vi "Curtin1_NewTest.vi"(9 "Template name":string, 11 "Settings":T2={"Name of test"="", "Date"=timestamp(0 s since 1904-01-01), "Location"="", "Default Template"="", "Soundcard"="", "resolution"=32, "Sampling rate"=48000, "Ch1 Gain "=25.0, "Ch2 Gain"=10.0, "Sample time (s)"=0.3, "Pre-trigger (s)"=0.01, "Hammer Threshold"=10.0, "Positions"=12, "Taps/Position"=5, "Set Names"="", "Freq resolution"=10.0, "Hammer cutoff"=0.0, "Mic cutoff"=0.0, "Double bounce "=0.0, "Hammer Cal"=10.0, "dB Offset"=0.0, "Accel Cal"=10.0, "Vibrometer Cal"=0.0, "Mic Cal"=0.0, "Output"=2, "Voltage Cal"=0.01, "Vibrometer Port"="ASRL27::INSTR", "Range"=4, "High Pass"=2, "Bandwidth"=4, "X Range"=[{"Minimum"=200.0, "Maximum"=10000.0, "Increment"=10.0, "Minor Increment"=100.0, "Start"=200.0}, {"Minimum"=0.0, "Maximum"=0.05, "Increment"=0.025, "Minor Increment"=0.0025, "Start"=0.0}, {"Minimum"=0.0, "Maximum"=0.3, "Increment"=0.1, "Minor Increment"=0.01, "Start"=0.0}, {"Minimum"=200.0, "Maximum"=10000.0, "Increment"=10.0, "Minor Increment"=100.0, "Start"=1000.0}], "Y Range"=[{"Minimum"=-25.0, "Maximum"=0.0, "Increment"=5.0, "Minor Increment"=1.0, "Start"=-25.0}, {"Minimum"=-0.01, "Maximum"=0.1, "Increment"=0.02, "Minor Increment"=0.005, "Start"=0.0}, {"Minimum"=-0.1, "Maximum"=0.1, "Increment"=0.05, "Minor Increment"=0.01, "Start"=-0.1}, {"Minimum"=-35.0, "Maximum"=5.0, "Increment"=2.0, "Minor Increment"=0.5, "Start"=-34.0}], "dB Spread"=0.0, "Trigger"=0, "Ch_1"=25, "Ch_2"=25, "flip?"=FALSE, "60Hz"=FALSE, "Time Offset"=0.0, "Piezo Cal"=0.0, "Default Notes"=""} {"Ch_2" min=1 step=1; "Ch_1" min=1 max=100 step=1; "Trigger" items=["Hammer (force)", "Self-tap", "Spacebar"]; "Bandwidth" items=["1 kHz"=1, "5 kHz"=5, "10 kHz"=10, "25 kHz"=25, "50 kHz"=50, "100 kHz"=100]; "High Pass" items=["Off", "13 Hz", "104 Hz"]; "Range" items=["10 mm/s"=1, "20 mm/s"=2, "50 mm/s"=5, "100 mm/s"=10, "200 mm/s"=20, "500 mm/s"=50, "1 m/s"=100, "2 m/s"=200]; "Output" items=["Accelerometer", "Speed (from acceleration)", "Microphone", "Vibrometer"]; "Voltage Cal" format="%#_13g"; "Ch2 Gain" format="%#_13g"; "Ch1 Gain" format="%#_13g"; "Double bounce" min=0.0; "Mic cutoff" min=0.0 format="%#_4g"; "Hammer cutoff" min=0.0 format="%#_4g"; "Freq resolution" min=0.0; "Pre-trigger (s)" format="%#_13g"; "Date" format="%<%H:%M\n%d/%m/%y>T"; "resolution" items=["16 bit"=16, "24 bit"=24, "32 bit"=32]; "Sampling rate" items=["22050 samp/s"=22050, "44100 samp/s"=44100, "48000 samp/s"=48000]}) -> (2 "Success":bool, 3 "Settings Out":T1={"Name of test"="", "Date"=timestamp(0 s since 1904-01-01), "Location"="", "Template"="", "Soundcard"="", "resolution"=32, "Sampling rate"=48000, "Ch1 Gain "=25.0, "Ch2 Gain"=10.0, "Sample time (s)"=0.3, "Pre-trigger (s)"=0.01, "Hammer Threshold"=10.0, "Positions"=12, "Taps/Position"=5, "Set Names"="", "Freq resolution"=10.0, "Hammer cutoff"=0.0, "Mic cutoff"=0.0, "Double bounce "=0.0, "Hammer Cal"=10.0, "dB Offset"=0.0, "Accel Cal"=10.0, "Vibrometer Cal"=0.0, "Mic Cal"=0.0, "Output"=2, "Voltage Cal"=0.01, "Vibrometer Port"="ASRL27::INSTR", "Range"=4, "High Pass"=2, "Bandwidth"=4, "X Range"=[], "Y Range"=[], "dB Spread"=0.0, "Trigger"=0, "Ch_1"=25, "Ch_2"=25, "flip?"=FALSE, "60Hz"=FALSE, "Time offset"=0.0, "Piezo Cal"=1.0, "Default Notes"=""} {"Ch_2" min=1 step=1; "Ch_1" min=1 max=100 step=1; "Trigger" items=["Hammer (force)", "Self-tap", "Spacebar"]; "Bandwidth" items=["1 kHz"=1, "5 kHz"=5, "10 kHz"=10, "25 kHz"=25, "50 kHz"=50, "100 kHz"=100]; "High Pass" items=["Off", "13 Hz", "104 Hz"]; "Range" items=["10 mm/s"=1, "20 mm/s"=2, "50 mm/s"=5, "100 mm/s"=10, "200 mm/s"=20, "500 mm/s"=50, "1 m/s"=100, "2 m/s"=200]; "Output" items=["Accelerometer", "Speed (from acceleration)", "Microphone", "Vibrometer", "Piezo"]; "Voltage Cal" format="%#_13g"; "Ch2 Gain" format="%#_13g"; "Ch1 Gain" format="%#_13g"; "Double bounce" min=0.0; "Mic cutoff" min=0.0 format="%#_4g"; "Hammer cutoff" min=0.0 format="%#_4g"; "Freq resolution" min=0.0; "Pre-trigger (s)" format="%#_13g"; "Date" format="%<%H:%M\n%d/%m/%y>T"; "resolution" items=["16 bit"=16, "24 bit"=24, "32 bit"=32]; "Sampling rate" items=["22050 samp/s"=22050, "44100 samp/s"=44100, "48000 samp/s"=48000]})   [LabVIEW 2022 SP3]
uses:
  PreferencesControl.ctl
  <vilib>/Utility/miscctls.llb/LVSelectionTypeDef.ctl
  <vilib>/Utility/error.llb/Trim Whitespace One-Sided.vi
  Mic/Mic_Global.vi
panel:
  in  "View":bool
  out "Comparison info":string
  out "String":string="Updating Vibrometer..."
  out "start":T1={"Name of test"="", "Date"=timestamp(0 s since 1904-01-01), "Location"="", "Template"="", "Soundcard"="", "resolution"=0, "Sampling rate"=0, "Ch1 Gain "=25.0, "Ch2 Gain"=10.0, "Sample time (s)"=0.0, "Pre-trigger (s)"=0.0, "Hammer Threshold"=0.0, "Positions"=0, "Taps/Position"=0, "Set Names"="", "Freq resolution"=0.0, "Hammer cutoff"=0.0, "Mic cutoff"=0.0, "Double bounce "=0.0, "Hammer Cal"=0.0, "dB Offset"=0.0, "Accel Cal"=0.0, "Vibrometer Cal"=0.0, "Mic Cal"=0.0, "Output"=0, "Voltage Cal"=1.0, "Vibrometer Port"="ASRL27::INSTR", "Range"=4, "High Pass"=2, "Bandwidth"=4, "X Range"=[], "Y Range"=[], "dB Spread"=0.0, "Trigger"=0, "Ch_1"=25, "Ch_2"=25, "flip?"=FALSE, "60Hz"=FALSE, "Time offset"=0.0, "Piezo Cal"=1.0, "Default Notes"=""} {"Ch_2" min=1 step=1; "Ch_1" min=1 max=100 step=1; "Trigger" items=["Hammer (force)", "Self-tap", "Spacebar"]; "Bandwidth" items=["1 kHz"=1, "5 kHz"=5, "10 kHz"=10, "25 kHz"=25, "50 kHz"=50, "100 kHz"=100]; "High Pass" items=["Off", "13 Hz", "104 Hz"]; "Range" items=["10 mm/s"=1, "20 mm/s"=2, "50 mm/s"=5, "100 mm/s"=10, "200 mm/s"=20, "500 mm/s"=50, "1 m/s"=100, "2 m/s"=200]; "Output" items=["Accelerometer", "Speed (from acceleration)", "Microphone", "Vibrometer", "Piezo"]; "Voltage Cal" format="%#_13g"; "Ch2 Gain" format="%#_13g"; "Ch1 Gain" format="%#_13g"; "Double bounce" min=0.0; "Mic cutoff" min=0.0 format="%#_4g"; "Hammer cutoff" min=0.0 format="%#_4g"; "Freq resolution" min=0.0; "Pre-trigger (s)" format="%#_13g"; "Date" format="%<%H:%M\n%d/%m/%y>T"; "resolution" items=["16 bit"=16, "24 bit"=24, "32 bit"=32]; "Sampling rate" items=["22050 samp/s"=22050, "44100 samp/s"=44100, "48000 samp/s"=48000]}
  in  "DAQ":bool
  out "current":string
  out "Hammer Spectrum":cluster{dbl, "df":dbl, "FFT {X}":dbl[]}[](graph)=[{0.0, "df"=1.0, "FFT {X}"=array[24000 elements]}, {0.0, "df"=40000.0, "FFT {X}"=[-20.0, -20.0]}]
  out "Hammer Data":cluster{dbl, "dt":dbl, "Y":dbl[]}[](graph)=[{0.0, "dt"=2.0833333333333333e-05, "Y"=array[14400 elements]}, {0.0, "dt"=0.0, "Y"=[]}]
  out "Microphone Data":cluster{dbl, "dt":dbl, "Y":dbl[]}[](graph)=[{0.0, "dt"=2.0833333333333333e-05, "Y"=array[14400 elements]}, {0.0, "dt"=0.0, "Y"=[]}]
  out "Average FRF":cluster{dbl, "df":dbl, dbl[]}[](graph)=[{0.0, "df"=1.0, array[24000 elements]}, {0.0, "df"=1.0, array[24000 elements]}]
  out "Vib Cover":bool
  in  "Vibrometer 2":bool
  in  "Vibrometer":bool
  in  "Save as a Template":bool
  in  "Import Template":bool
  in  "Test":bool
  in  "device:":u16(ring) items=["BuerginBase Microphone", "485B39 200083408035100798118210422", "MacBook Pro Microphone", "Reincubate", "Microsoft Teams Audio", "Jump Desktop Microphone", "Jump Desktop Audio", "ZoomAudioDevice"]
  in  "OK Button":bool
  in  "Cancel Button":bool
  in  "Instrument Notes":string
  in  "Tag List":bool
  in  "Instrument Name":string(combo)
  in  "Instrument Keywords":string
  out "File name":string
  in  "Test Name":string
  in  "Import Calib":bool
  # "New Test"
  # "Adjust default scale ranges"
  # "Adjust default scale ranges"
  # "Hz"
  # "dB"
  # "dB"
  # "sec"
  # "sec"
  # "mV/Pa"
  # "mV/m/s2"
  # "mV/mm/s"
  # "V/N"
  # "sec"
  # "sec"
  # "mV/N"
  # "a.u."
  # "a.u."
  # "sec"
  # "mV/Pa"
  # "mV/m/s2"
  # "mV/mm/s"
  # "V/N"
  # "sec"
  # "sec"
  # "mV/N"
  # "Hz"
  # "a.u."
  # "dB"
  # "a.u."
  # "dB"
  # "sec"
  # "sec"
  # "sec"
  # "Hz"
  # "dB"
  # "dB"
  # "sec"
  # "sec"
  # "mV/Pa"
  # "mV/m/s2"
  # "mV/mm/s"
  # "V/N"
  # "sec"
  # "sec"
  # "mV/N"
  # "a.u."
  # "a.u."
  # "sec"
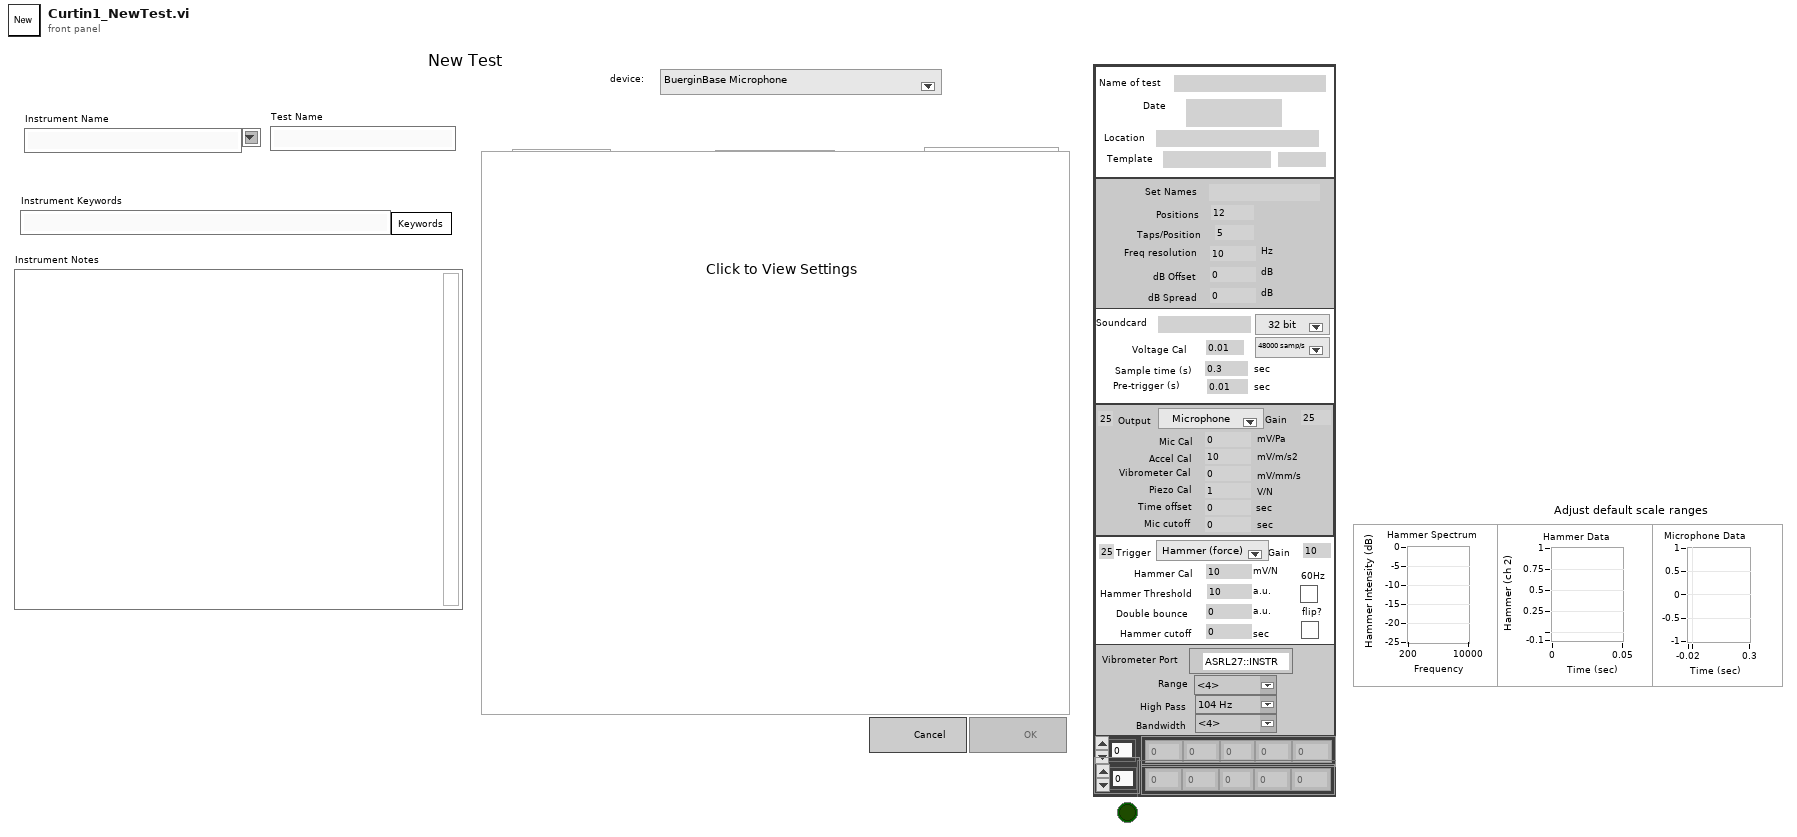
[diagram p1: front panel]
types:
  T1 = typedef "PreferencesControl.ctl" = cluster{"Name of test":string, "Date":timestamp, "Location":string, "Template":string, "Soundcard":string, "resolution":u16, "Sampling rate":u16, "Ch1 Gain ":dbl, "Ch2 Gain":dbl, "Sample time (s)":dbl, "Pre-trigger (s)":dbl, "Hammer Threshold":dbl, "Positions":i16, "Taps/Position":i16, "Set Names":string, "Freq resolution":dbl, "Hammer cutoff":dbl, "Mic cutoff":dbl, "Double bounce ":dbl, "Hammer Cal":dbl, "dB Offset":dbl, "Accel Cal":dbl, "Vibrometer Cal":dbl, "Mic Cal":dbl, "Output":u16, "Voltage Cal":dbl, "Vibrometer Port":refnum<visa-resource-name>, "Range":u16, "High Pass":u16, "Bandwidth":u16, "X Range":cluster{"Minimum":dbl, "Maximum":dbl, "Increment":dbl, "Minor Increment":dbl, "Start":dbl}[], "Y Range":cluster{"Minimum":dbl, "Maximum":dbl, "Increment":dbl, "Minor Increment":dbl, "Start":dbl}[], "dB Spread":dbl, "Trigger":u16, "Ch_1":u8, "Ch_2":u8, "flip?":bool, "60Hz":bool, "Time offset":dbl, "Piezo Cal":dbl, "Default Notes":string}
  T2 = cluster{"Name of test":string, "Date":timestamp, "Location":string, "Default Template":string, "Soundcard":string, "resolution":u16, "Sampling rate":u16, "Ch1 Gain ":dbl, "Ch2 Gain":dbl, "Sample time (s)":dbl, "Pre-trigger (s)":dbl, "Hammer Threshold":dbl, "Positions":i16, "Taps/Position":i16, "Set Names":string, "Freq resolution":dbl, "Hammer cutoff":dbl, "Mic cutoff":dbl, "Double bounce ":dbl, "Hammer Cal":dbl, "dB Offset":dbl, "Accel Cal":dbl, "Vibrometer Cal":dbl, "Mic Cal":dbl, "Output":u16, "Voltage Cal":dbl, "Vibrometer Port":refnum<visa-resource-name>, "Range":u16, "High Pass":u16, "Bandwidth":u16, "X Range":cluster{"Minimum":dbl, "Maximum":dbl, "Increment":dbl, "Minor Increment":dbl, "Start":dbl}[], "Y Range":cluster{"Minimum":dbl, "Maximum":dbl, "Increment":dbl, "Minor Increment":dbl, "Start":dbl}[], "dB Spread":dbl, "Trigger":u16, "Ch_1":u8, "Ch_2":u8, "flip?":bool, "60Hz":bool, "Time Offset":dbl, "Piezo Cal":dbl, "Default Notes":string}
  T3 = enum8{"Enabled", "Disabled", "Disabled and Grayed Out"}
  T4 = typedef "LVSelectionTypeDef.ctl" = cluster{"Selection Start":u32, "Selection End":u32}
  T5 = typedef "LVRangeTypeDef.ctl" = cluster{"Minimum":dbl, "Maximum":dbl, "Increment":dbl, "Minor Increment":dbl, "Start":dbl}
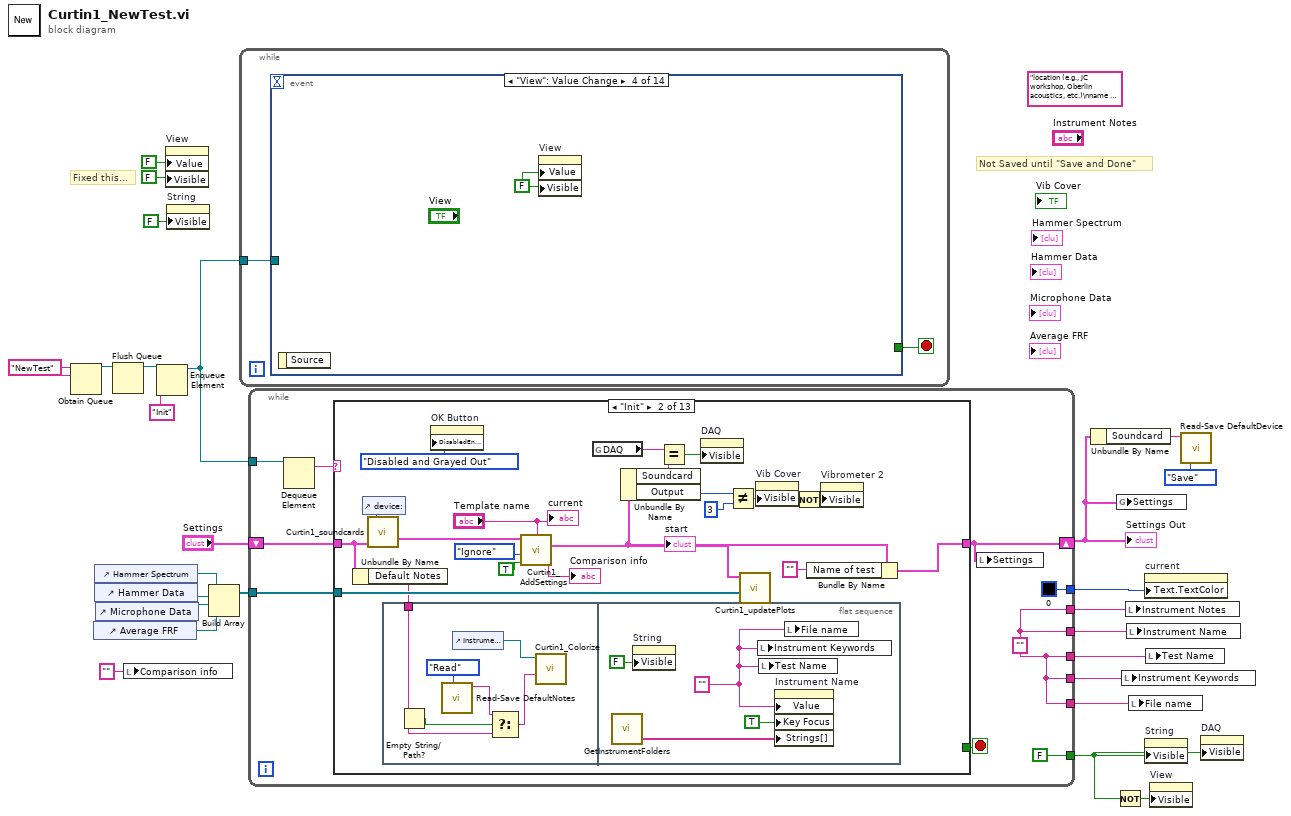
[diagram p0: block diagram]
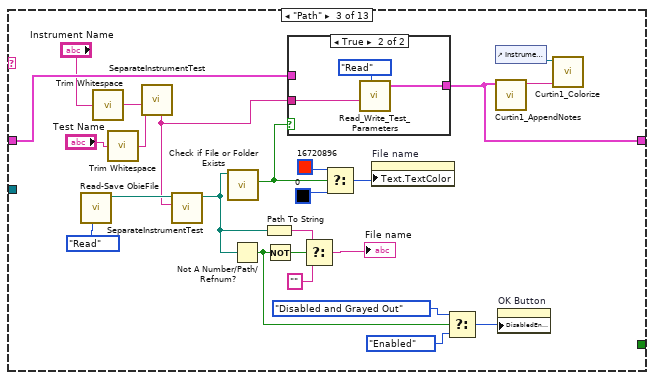
[diagram p3: hidden frame]
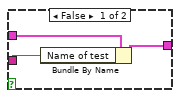
[diagram p4: hidden frame]
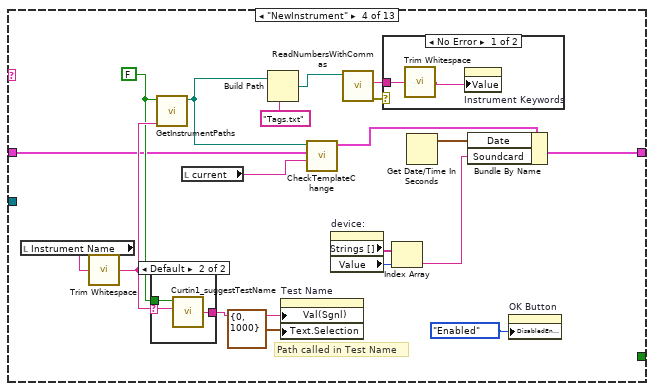
[diagram p5: hidden frame]
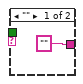
[diagram p7: hidden frame]
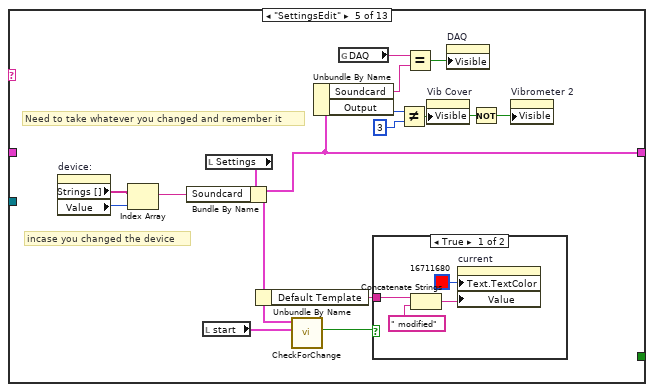
[diagram p8: hidden frame]
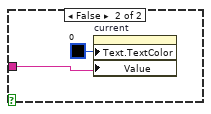
[diagram p9: hidden frame]
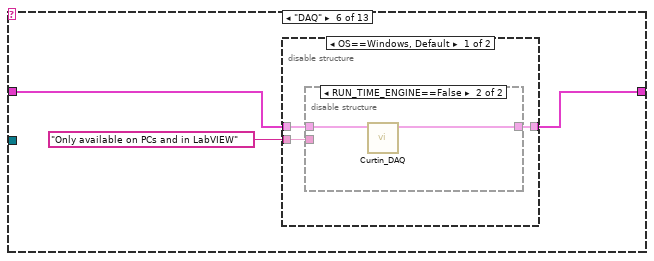
[diagram p10: hidden frame]
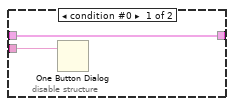
[diagram p11: hidden frame]
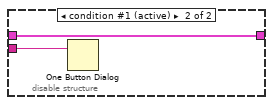
[diagram p12: hidden frame]
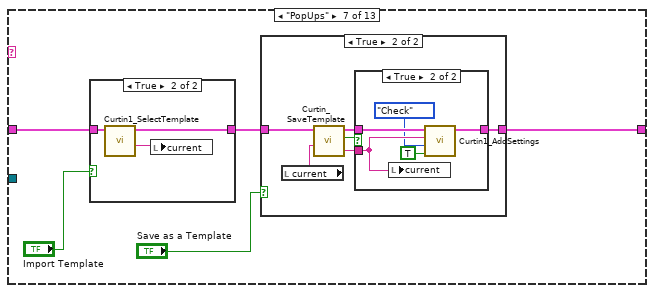
[diagram p13: hidden frame]
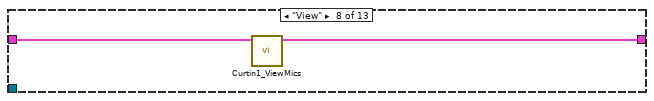
[diagram p17: hidden frame]
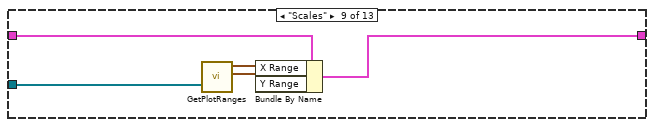
[diagram p18: hidden frame]
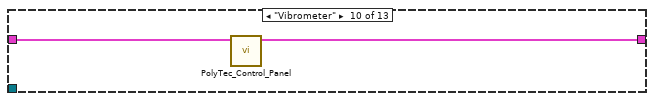
[diagram p19: hidden frame]
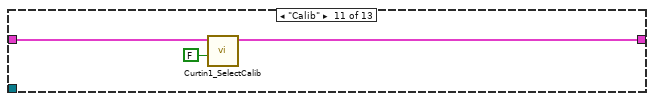
[diagram p20: hidden frame]
diagram:
  (unwired) "location (e.g., JC workshop, Oberlin acoustics, etc.)\nname of experiment (if applicable) \nnames of researchers\n\nInstrument Information:\ninstrument (e.g., violin, viola, cello, guitar, mandolin, etc.) \nmodel (e.g., Titian Strad, Guadagnini, personal, etc.) \nmaker name\nmaker ID (e.g., serial number)\nyear built (4 digits)\ncountry of origin \nsession (e.g. Oberlin 2017, VSA 2008) \nmaking school (e.g. Old Italian) \n\nMeasurement Information:\ntype (Radiation, admittance, modal analysis, taptones, etc.) \nprotocol (HV24, etc.)\n" ("Notes")
  w26 = "NewTest" ("name (unnamed)")
  # "Fixed this..."
  # "Not Saved until \"Save and Done\""
  n1 = Obtain Queue(name (unnamed)=w26, element data type=w26) -> (queue out=w3:refnum<queue>)  [unwired: 3 in, 2 out]
  n2 = control-ref of="Average FRF"() -> (w14:refnum<vi>)
  n3 = control-ref of="Hammer Spectrum"() -> (w17:refnum<vi>)
  n4 = control-ref of="Hammer Data"() -> (w16:refnum<vi>)
  n5 = control-ref of="Microphone Data"() -> (w15:refnum<vi>)
  n6 = Flush Queue(queue=w3) -> (queue out=w2:refnum<queue>)  [unwired: 1 in, 2 out]
  n7 = local write "Comparison info"("" ("Comparison info")) -> ()
  n8 = Enqueue Element(queue=w2, element="Init") -> (queue out=w24:refnum<queue>)  [unwired: 2 in, 2 out]
  n9 = property on="View" class="Bool (strict)"("Value"=FALSE ("View"), "Visible"=FALSE) -> ()  [unwired: 2 in, 2 out]
  n10 = property on="String" class="Str"("Visible"=FALSE) -> ()  [unwired: 2 in, 2 out]
  n11 = Build Array(w17, w16, w15, w14) -> (w13:refnum<vi>[])
  n12 = while {
    tunnel: w24 -> [w27]
    stop <- w28 stop-if-true
    n13 = event shown="[3] \"View\": Value Change" {
      selector: _ -> [_ _ _ _ _ _ _ _ _ _ _ _ _ _]
      dyn-events: _ -> [_ _ _ _ _ _ _ _ _ _ _ _ _ _]
      timeout: _ -> [_ _ _ _ _ _ _ _ _ _ _ _ _ _]
      tunnel: [_ _ _ _ _ _ _ _ _ _ _ _ TRUE _] -> w28
      tunnel: w27 -> [_ w29 w31 _ w34 w36 w38 w40 w42 w44 w46 w48 w54 _]
      event Timeout {
        n14 = event-data() -> ()  [unwired: 1 in, 3 out]
      }
      event "Test Name": Value Change {
        n15 = event-data() -> ()  [unwired: 1 in, 1 out]
        n16 = Enqueue Element(queue=w29, element="Path") -> ()  [unwired: 2 in, 3 out]
      }
      event "Settings": Value Change {
        n17 = event-data() -> ()  [unwired: 1 in, 1 out]
        n18 = Enqueue Element(queue=w31, element="SettingsEdit") -> ()  [unwired: 2 in, 3 out]
      }
      event "View": Value Change {
        w33 = FALSE ("Visible")
        n19 = event-data() -> ()  [unwired: 1 in, 1 out]
        n20 = property on="View" class="Bool (strict)"("Value"=w33, "Visible"=w33) -> ()  [unwired: 2 in, 2 out]
      }
      event "Instrument Name": Value Change {
        n21 = event-data() -> ()  [unwired: 1 in, 6 out]
        n22 = Enqueue Element(queue=w34, element="NewInstrument") -> ()  [unwired: 2 in, 3 out]
      }
      event "device:": Value Change {
        n23 = event-data() -> ()  [unwired: 1 in, 6 out]
        n24 = Enqueue Element(queue=w36, element="SettingsEdit") -> ()  [unwired: 2 in, 3 out]
      }
      event "DAQ": Value Change {
        n25 = event-data() -> ()  [unwired: 1 in, 6 out]
        n26 = Enqueue Element(queue=w38, element="DAQ") -> ()  [unwired: 2 in, 3 out]
      }
      event "Import Calib": Value Change {
        n27 = event-data() -> ()  [unwired: 1 in, 6 out]
        n28 = Enqueue Element(queue=w40, element="Calib") -> ()  [unwired: 2 in, 3 out]
      }
      event "Import Template", "Save as a Template": Value Change {
        n29 = event-data() -> ()  [unwired: 1 in, 1 out]
        n30 = Enqueue Element(queue=w42, element="PopUps") -> ()  [unwired: 2 in, 3 out]
      }
      event "Test": Value Change {
        n31 = event-data() -> ()  [unwired: 1 in, 6 out]
        n32 = Enqueue Element(queue=w44, element="View") -> ()  [unwired: 2 in, 3 out]
      }
      event "Average FRF", "Microphone Data", "Hammer Data", "Hammer Spectrum": Scale Range Change {
        n33 = event-data() -> ()  [unwired: 1 in, 8 out]
        n34 = Enqueue Element(queue=w46, element="Scales") -> ()  [unwired: 2 in, 3 out]
      }
      event "Vibrometer", "Vibrometer 2": Value Change {
        n35 = event-data() -> ()  [unwired: 1 in, 6 out]
        n36 = Enqueue Element(queue=w48, element="Vibrometer") -> ()  [unwired: 2 in, 3 out]
      }
      event Panel Close; "OK Button", "Cancel Button": Value Change {
        n37 = event-data() -> ()  [unwired: 1 in, 1 out]
        n38 = Select(t="Save and Done" ("element"), s="OK Button", f="Done" ("element")) -> (s? t:f=w51:string)
        n39 = Enqueue Element(queue=w54, element=w51) -> ()  [unwired: 2 in, 3 out]
        "Success" <- "OK Button"
      }
      event "Tag List", "Instrument Keywords": Value Change {
        n40 = event-data() -> ()  [unwired: 1 in, 1 out]
        n41 = case shown="True" "Tag List" {
          tunnel: ["" ("Tags out") w71] -> w60
          frame False {
          }
          frame True {
            n42 = call "RequestTags.vi"() -> ("Tags out"=w71:string)  [unwired: 11 in]
          }
        }
        n43 = case shown="Default" "Instrument Keywords" {
          tunnel: w60 -> [w61 w62]
          tunnel: "Instrument Keywords" -> [_ w64]
          tunnel: [w61 w63] -> w58
          frame "" {
          }
          frame Default {
            n44 = case shown="Default" w62 {
              selector: w62 -> [_ w66]
              tunnel: w64 -> [w65 w69]
              tunnel: [w65 w68] -> w63
              frame "" {
              }
              frame Default {
                n45 = Concatenate Strings(w69, "," ("string"), w66) -> (w68:string)
              }
            }
          }
        }
        n46 = call "RemoveDuplicateTags.vi"("Tags"=w58) -> ("Tag string"=w56:string)  [unwired: 9 in, 1 out]
        n47 = local write "Instrument Keywords"(w56) -> ()
      }
    }
  }
  n48 = while {
    tunnel: w24 -> [w79]
    shift-right: [w72] -> w5
    shift-left: "Settings" -> [w77]
    tunnel: [w76] -> w23
    tunnel: [w76] -> w22
    tunnel: [w76] -> w21
    tunnel: [w76] -> w20
    tunnel: [w76] -> w19
    tunnel: [FALSE ("Visible")] -> w8
    tunnel: w13 -> [w74]
    tunnel: [u32 0 ("Text.Text Colors:Text Color")] -> w12
    stop <- w78 stop-if-true
    w76 = "" ("Value (Signaling)")
    n49 = Dequeue Element(queue=w79) -> (element=w80:string)  [unwired: 2 in, 3 out]
    n50 = case shown="\"Init\"" w80 {
      tunnel: [_ _ _ _ _ _ _ _ _ _ _ TRUE TRUE] -> w78
      tunnel: w77 -> [w81 w84 w119 w149 _ w189 w203 w223 w225 w230 w233 w234 w239]
      tunnel: [w81 w100 w116 w154 w172 w188 w200 w222 w224 w229 w232 w234 w236] -> w72
      tunnel: w74 -> [_ w87 _ _ _ _ _ _ w226 _ _ _ _]
      frame Default {
      }
      frame "Init" {
        n51 = Unbundle By Name(w84) -> ("Default Notes"=w83:string)
        n52 = control-ref of="device:"() -> (w101:refnum<vi>)
        n53 = call "Curtin1_soundcards.vi"("Settings In"=w84, "device:"=w101) -> ("Settings Out"=w85:T1)  [unwired: 8 in, 1 out]
        n54 = flat-sequence {
          tunnel: w83 -> [w103]
          frame #0 {
            n55 = Empty String/Path?(string/path=w103) -> (empty?=w102:bool)
            n56 = call "Read-Save DefaultNotes.vi"("Task"=enum16{"Save", "Read"}."Read") -> ("Notes Out"=w105:string)  [unwired: 9 in, 1 out]
            n57 = control-ref of="Instrument Notes"() -> (w106:refnum<vi>)
            n58 = Select(t=w105, s=w102, f=w103) -> (s? t:f=w104:string)
            n59 = call "Curtin1_Colorize.vi"("Instrument Notes"=w104, "Text"=w106) -> ()  [unwired: 10 in]
          }
          frame #1 {
            w109 = "" ("Value (Signaling)")
            n60 = call "GetInstrumentFolders.vi"() -> ("folder names"=w111:string[])  [unwired: 11 in]
            n61 = property on="String" class="Str"("Visible"=FALSE) -> ()  [unwired: 2 in, 2 out]
            n62 = local write "Instrument Keywords"(w109) -> ()
            n63 = local write "Test Name"(w109) -> ()
            n64 = property on="Instrument Name" class="CmbBox"("Value"=w109, "Key Focus"=TRUE, "Strings[]"=w111) -> ()  [unwired: 2 in, 2 out]
            n65 = local write "File name"(w109) -> ()
          }
        }
        n66 = property on="OK Button" class="Bool"("DisabledEnum"=T3."Disabled and Grayed Out" ("Disabled")) -> ()  [unwired: 2 in, 2 out]
        n67 = call "Curtin1_AddSettings.vi"("Date?"=TRUE, "Check?"=enum16{"Ignore", "Check", "Replace"}."Ignore", "Template"="Template name", "Settings in"=w85) -> ("text"=→"Comparison info":string, "Settings Out"=w86:T1)  [unwired: 6 in]
        "start" <- w86
        n68 = global read "Mic_Global.vi" "DAQ"() -> (w93:string)
        n69 = Unbundle By Name(w86) -> ("Soundcard"=w92:string, "Output"=w98:u16)
        n70 = Equal?(x=w93, y=w92) -> (x = y?=w91:bool)
        n71 = property on="DAQ" class="Bool"("Visible"=w91) -> ()  [unwired: 2 in, 2 out]
        n72 = Not Equal?(x=w98, y=u16 3) -> (x != y?=w96:bool)
        n73 = call "Curtin1_updatePlots.vi"("plots"=w87, "Settings"=w86) -> ()  [unwired: 10 in]
        n74 = property on="Vib Cover" class="Bool (strict)"("Visible"=w96) -> ()  [unwired: 2 in, 2 out]
        n75 = Not(x=w96) -> (.not. x?=w95:bool)
        n76 = Bundle By Name(cluster=w86, "Name of test"="") -> (w100:T1)
        n77 = property on="Vibrometer 2" class="Bool"("Visible"=w95) -> ()  [unwired: 2 in, 2 out]
        "current" <- "Template name"
      }
      frame "Path" {
        n78 = call "Read-Save ObieFile.vi"("Task"=enum16{"Save", "Read"}."Read") -> ("DataPath Out"=w122:path)  [unwired: 8 in, 2 out]
        n79 = call <vilib>:"Trim Whitespace.vi"("string"="Instrument Name") -> ("trimmed string"=w115:string)  [unwired: 1 in]
        n80 = call <vilib>:"Trim Whitespace.vi"("string"="Test Name") -> ("trimmed string"=w112:string)  [unwired: 1 in]
        n81 = call "SeparateInstrumentTest.vi"("test in"=w112, "Instrument in"=w115) -> ("Instrument -- test out"=w120:string)  [unwired: 5 in, 4 out]
        n82 = call "SeparateInstrumentTest.vi"("Instrument"=w120, "path in"=w122) -> ("path out"=w121:path)  [unwired: 5 in, 4 out]
        n83 = call <vilib>:"Check if File or Folder Exists.vi"("path"=w121) -> ("file or folder exists?"=w124:bool)  [unwired: 8 in, 2 out]
        n84 = Not A Number/Path/Refnum?(number/path/refnum=w121) -> (NaN/Path/Refnum?=w134:bool)
        n85 = Path To String(path=w121) -> (string=w133:string)
        n86 = Not(x=w134) -> (.not. x?=w132:bool)
        n87 = case shown="True" w124 {
          tunnel: w119 -> [w138 _]
          tunnel: [w137 w139] -> w116
          tunnel: w120 -> [w136 w140]
          frame False {
            n88 = Bundle By Name(cluster=w138, "Name of test"=w136) -> (w137:T1)
          }
          frame True {
            n89 = call "Read_Write_Test_Parameters.vi"("Task"=enum16{"Save", "Read", "Clear"}."Read", "Instrument Name"=w140) -> ("Settings"=w139:T1)  [unwired: 8 in, 1 out]
          }
        }
        n90 = Select(t=w133, s=w132, f="") -> (s? t:f=→"File name":string)
        n91 = Select(t=u32 16720896, s=w124, f=u32 0) -> (s? t:f=w131:u32)
        n92 = property on="File name" class="Str"("Text.TextColor"=w131) -> ()  [unwired: 2 in, 2 out]
        n93 = Select(t=T3."Disabled and Grayed Out" ("Disabled"), s=w134, f=T3."Enabled" ("Disabled")) -> (s? t:f=w135:T3)
        n94 = control-ref of="Instrument Notes"() -> (w118:refnum<vi>)
        n95 = call "Curtin1_AppendNotes.vi"("Settings"=w116) -> ("Instrument Notes"=w117:string)  [unwired: 10 in]
        n96 = property on="OK Button" class="Bool"("DisabledEnum"=w135) -> ()  [unwired: 2 in, 2 out]
        n97 = call "Curtin1_Colorize.vi"("Instrument Notes"=w117, "Text"=w118) -> ()  [unwired: 10 in]
      }
      frame "NewInstrument" {
        w151 = FALSE ("Build?")
        # "Path called in Test Name"
        n98 = local read "Instrument Name"() -> (w157:string)
        n99 = call <vilib>:"Trim Whitespace.vi"("string"=w157) -> ("trimmed string"=w155:string)  [unwired: 1 in]
        n100 = case shown="Default" w155 {
          selector: w155 -> [_ w166]
          tunnel: ["" w165] -> w160
          tunnel: w151 -> [_ w164]
          frame "" {
          }
          frame Default {
            n101 = call "Curtin1_suggestTestName.vi"("instrument"=w166, "Build?"=w164) -> ("Suggested Test"=w165:string)  [unwired: 9 in]
          }
        }
        n102 = call "GetInstrumentPaths.vi"("Instrument"=w155, "Build?"=w151) -> ("Path To Instrument Folder"=w156:path)  [unwired: 5 in, 4 out]
        n103 = local read "current"() -> (w145:string)
        n104 = Build Path(base path=w156, name or relative path="Tags.txt") -> (appended path=w144:path)
        n105 = property on="Test Name" class="Str"("Val(Sgnl)"=w160, "Text.Selection"=T4 {"Selection Start"=0, "Selection End"=1000}) -> ()  [unwired: 2 in, 2 out]
        n106 = call "CheckTemplateChange.vi"("Template"=w145, "Settings In"=w149, "Path To Instrument Folder"=w156) -> ("Settings  Out"=w146:T1)  [unwired: 7 in, 1 out]
        n107 = property on="device:" class="Ring (strict)"() -> ("Strings []"=w152:string[], "Value"=w153:u16)  [unwired: 2 in, 2 out]
        n108 = call "ReadNumbersWithCommas.vi"("file (use dialog)"=w144) -> ("error out"=w142:errorcluster, "text"=w143:string)  [unwired: 7 in, 2 out]
        n109 = case shown="No Error" w142 {
          tunnel: w143 -> [w162 _]
          frame No Error {
            n110 = call <vilib>:"Trim Whitespace.vi"("string"=w162) -> ("trimmed string"=w161:string)  [unwired: 1 in]
            n111 = property on="Instrument Keywords" class="Str"("Value"=w161) -> ()  [unwired: 2 in, 2 out]
          }
          frame Error {
          }
        }
        n112 = Index Array(array=w152, index=w153) -> (element=w148:string)
        n113 = Get Date/Time In Seconds() -> (seconds since 1Jan1904=w147:timestamp)
        n114 = Bundle By Name(cluster=w146, "Date"=w147, "Soundcard"=w148) -> (w154:T1)
        n115 = property on="OK Button" class="Bool"("DisabledEnum"=T3."Enabled" ("Disabled")) -> ()  [unwired: 2 in, 2 out]
      }
      frame "SettingsEdit" {
        # "incase you changed the device"
        # "Need to take whatever you changed and remember it"
        n116 = property on="device:" class="Ring (strict)"() -> ("Strings []"=w180:string[], "Value"=w181:u16)  [unwired: 2 in, 2 out]
        n117 = Index Array(array=w180, index=w181) -> (element=w178:string)
        n118 = local read "start"() -> (w167:T1)
        n119 = local read "Settings"() -> (w179:T2)
        n120 = Bundle By Name(cluster=w179, "Soundcard"=w178) -> (w172:T2)
        n121 = Unbundle By Name(w172) -> ("Default Template"=w173:string)
        n122 = call "CheckForChange.vi"("Original Settings"=w167, "Current Settings"=w172) -> ("change?"=w171:bool)  [unwired: 8 in, 1 out]
        n123 = Unbundle By Name(w172) -> ("Soundcard"=w168:string, "Output"=w177:u16)
        n124 = global read "Mic_Global.vi" "DAQ"() -> (w170:string)
        n125 = case shown="True" w171 {
          tunnel: w173 -> [w182 w186]
          frame True {
            n126 = Concatenate Strings(w182, " modified" ("string")) -> (w183:string)
            n127 = property on="current" class="Str"("Text.TextColor"=u32 16711680 ("Text.Text Colors:Text Color"), "Value"=w183) -> ()  [unwired: 2 in, 2 out]
          }
          frame False {
            n128 = property on="current" class="Str"("Text.TextColor"=u32 0 ("Text.Text Colors:Text Color"), "Value"=w186) -> ()  [unwired: 2 in, 2 out]
          }
        }
        n129 = Not Equal?(x=w177, y=u16 3) -> (x != y?=w176:bool)
        n130 = Equal?(x=w170, y=w168) -> (x = y?=w169:bool)
        n131 = property on="Vib Cover" class="Bool (strict)"("Visible"=w176) -> ()  [unwired: 2 in, 2 out]
        n132 = property on="DAQ" class="Bool"("Visible"=w169) -> ()  [unwired: 2 in, 2 out]
        n133 = Not(x=w176) -> (.not. x?=w174:bool)
        n134 = property on="Vibrometer 2" class="Bool"("Visible"=w174) -> ()  [unwired: 2 in, 2 out]
      }
      frame "DAQ" {
        n135 = disable-structure shown="OS==Windows, Default" {
          disable-tunnel: "Only available on PCs and in LabVIEW" ("message") -> [w193 w199]
          disable-tunnel: w189 -> [w192 w198]
          disable-tunnel: [w191 w198] -> w188
          frame condition #0 {
            n136 = disable-structure shown="RUN_TIME_ENGINE==False" {
              disable-tunnel: w193 -> [w195 _]
              disable-tunnel: w192 -> [w194 w197]
              disable-tunnel: [w194 w196] -> w191
              frame condition #0 {
                n137 = One Button Dialog(message=w195) -> ()  [unwired: 1 in, 1 out]
              }
              frame condition #1 (active) {
                n138 = call "Curtin_DAQ.vi"("Settings"=w197) -> ("Settings out"=w196:T1)  [unwired: 10 in]
              }
            }
          }
          frame condition #1 (active) {
            n139 = One Button Dialog(message=w199) -> ()  [unwired: 1 in, 1 out]
          }
        }
      }
      frame "PopUps" {
        n140 = case shown="True" "Import Template" {
          tunnel: w203 -> [w218 w221]
          tunnel: [w218 w219] -> w201
          frame False {
          }
          frame True {
            n141 = call "Curtin1_SelectTemplate.vi"("Settings in"=w221) -> ("New Template"=w220:string, "Settings out"=w219:T1)  [unwired: 9 in]
            n142 = local write "current"(w220) -> ()
          }
        }
        n143 = case shown="True" "Save as a Template" {
          tunnel: [w205 w207] -> w200
          tunnel: w201 -> [w205 w211]
          frame False {
          }
          frame True {
            n144 = local read "current"() -> (w206:string)
            n145 = call "Curtin_SaveTemplate.vi"("Template Name"=w206, "Settings in"=w211) -> ("New Template"=w208:string, "Good?"=w210:bool, "Settings out"=w209:T1)  [unwired: 7 in]
            n146 = case shown="True" w210 {
              tunnel: w209 -> [w212 w217]
              tunnel: w208 -> [_ w215]
              tunnel: [w212 w216] -> w207
              frame False {
              }
              frame True {
                n147 = local write "current"(w215) -> ()
                n148 = call "Curtin1_AddSettings.vi"("Date?"=TRUE, "Check?"=enum16{"Ignore", "Check", "Replace"}."Check", "Template"=w215, "Settings in"=w217) -> ("Settings Out"=w216:T1)  [unwired: 6 in, 1 out]
              }
            }
          }
        }
      }
      frame "View" {
        n149 = call "Curtin1_ViewMics.vi"("Settings"=w223) -> ("Settings Out"=w222:T1)  [unwired: 10 in]
      }
      frame "Scales" {
        n150 = call "GetPlotRanges.vi"("plots"=w226) -> ("Yscales"=w228:T5[], "Xscales"=w227:T5[])  [unwired: 9 in]
        n151 = Bundle By Name(cluster=w225, "X Range"=w227, "Y Range"=w228) -> (w224:T1)
      }
      frame "Vibrometer" {
        n152 = call "PolyTec_Control_Panel.vi"("Settings in"=w230) -> ("Settings Out"=w229:T1)  [unwired: 8 in, 2 out]
      }
      frame "Calib" {
        n153 = call "Curtin1_SelectCalib.vi"("Save?"=FALSE, "Settings in"=w233) -> ("Settings out"=w232:T1)  [unwired: 9 in]
      }
      frame "Done" {
      }
      frame "Save and Done" {
        n154 = local read "Instrument Keywords"() -> (w240:string)
        n155 = Get Date/Time In Seconds() -> (seconds since 1Jan1904=w243:timestamp)
        n156 = local read "Instrument Notes"() -> (w241:string)
        n157 = Bundle By Name(cluster=w239, "Date"=w243) -> (w237:T1)
        n158 = call "Read_Write_Test_Parameters.vi"("Task"=enum16{"Save", "Read", "Clear"}."Save", "Settings"=w237) -> ()  [unwired: 8 in, 2 out]
        n159 = call "Curtin1_SaveTagsFile.vi"("Tags"=w240, "Settings in"=w237) -> ()  [unwired: 10 in]
        n160 = call "Curtin1_SaveNotesFile.vi"("Notes"=w241, "Settings in"=w237) -> ()  [unwired: 10 in]
        n161 = call "Curtin1_SaveLastSettingsFile.vi"("Settings in"=w237) -> ()  [unwired: 11 in]
        n162 = Unbundle By Name(w237) -> ("Output"=w238:u16)
        n163 = case shown="3" w238 {
          tunnel: w237 -> [w245 w249]
          tunnel: [w245 w247] -> w236
          frame 0, Default {
          }
          frame 3 {
            n164 = call "OverallControl.vi"("Settings"=w249) -> ("Success?"=w250:bool, "VISA Refnum out"=w248:refnum<visa-resource-name>)  [unwired: 9 in]
            n165 = property on="String" class="Str"("Visible"=TRUE) -> ()  [unwired: 2 in, 2 out]
            n166 = case shown="True" w250 {
              tunnel: w249 -> [w251 w255]
              tunnel: w248 -> [_ w254]
              tunnel: [w251 w253] -> w247
              frame False {
                n167 = One Button Dialog(message="Vibrometer not responding") -> ()  [unwired: 1 in, 1 out]
              }
              frame True {
                n168 = Bundle By Name(cluster=w255, "Vibrometer Port"=w254) -> (w253:T1)
              }
            }
          }
        }
      }
    }
    n169 = local write "Settings"(w72) -> ()
  }
  "Settings Out" <- w5
  n170 = Unbundle By Name(w5) -> ("Soundcard"=w4:string)
  n171 = Not(x=w8) -> (.not. x?=w10:bool)
  n172 = global write "Mic_Global.vi" "Settings"(w5) -> ()
  n173 = local write "Instrument Keywords"(w20) -> ()
  n174 = local write "Instrument Notes"(w23) -> ()
  n175 = local write "Instrument Name"(w22) -> ()
  n176 = local write "File name"(w19) -> ()
  n177 = property on="current" class="Str"("Text.TextColor"=w12) -> ()  [unwired: 2 in, 2 out]
  n178 = property on="String" class="Str"("Visible"=w8) -> ()  [unwired: 2 in, 2 out]
  n179 = local write "Test Name"(w21) -> ()
  n180 = property on="View" class="Bool (strict)"("Visible"=w10) -> ()  [unwired: 2 in, 2 out]
  n181 = call "Read-Save DefaultDevice.vi"("Task"=enum16{"Save", "Read"}."Save", "Soundcard"=w4) -> ()  [unwired: 8 in, 2 out]
  n182 = property on="DAQ" class="Bool"("Visible"=w8) -> ()  [unwired: 2 in, 2 out]
